vi "Test VI 1.vi"() -> ()   [LabVIEW 2022 SP3]
doc: "Block Diagram 1\n\nLorem ipsum dolor sit amet, consectetur adipiscing elit. Pellentesque gravida dolor et ex feugiat finibus."
panel:
  out "VI Description":string
  # "Front Panel 1\n\nLorem ipsum dolor sit amet, consectetur adipiscing elit. Pellentesque gravida dolor et ex feugiat finibus."
  # "Front Panel 4\n\nLorem ipsum dolor sit amet, consectetur adipiscing elit. Fusce sed augue venenatis lacus tempor malesuada. Ut eget leo sed enim aliquam porta vel at lectus. Vestibulum pretium lacinia finibus. Ut rutrum tincidunt justo, quis accumsan mauris consectetur blandit. Pellentesque sodales urna ac elit pharetra imperdiet. Phasellus felis mi, mollis non elementum et, auctor sit amet ligula. Vivamus vel dictum mi.\n\nDonec tempus orci vitae quam venenatis gravida. Nunc consequat ligula placerat ante molestie iaculis. Integer condimentum eget sapien vel vulputate. Morbi placerat, nibh iaculis gravida luctus, neque magna sodales arcu, non pellentesque mauris dolor at neque. Quisque ut erat tellus. Pellentesque nec gravida diam. Aliquam in ligula augue. Cras in tortor a erat vehicula ullamcorper ut in nisl. Nam nunc turpis, finibus id gravida vitae, interdum in dolor. Vestibulum et libero mi. Nam rhoncus lorem vulputate sodales accumsan.\n\nPhasellus in porttitor urna. Donec sodales imperdiet tellus, at interdum dolor auctor vehicula. Nullam risus sem, tincidunt ullamcorper purus nec, sagittis pharetra sem. Suspendisse blandit mattis quam et tristique. Aenean interdum quam non ligula faucibus pretium in nec ante. Curabitur euismod enim ac faucibus facilisis. Sed sed nisl finibus eros venenatis ornare sit amet quis eros. Integer pellentesque non ligula eget gravida. Aenean fringilla tempus rutrum. Nulla ullamcorper vel lacus quis sodales. Curabitur vel porttitor arcu.\n\nNam in mi sagittis, pretium eros nec, hendrerit neque. Mauris volutpat sem ut eros ornare mattis. Pellentesque at feugiat turpis. Morbi ut diam eget eros fermentum pharetra. Phasellus dictum aliquet est, vel auctor nisi. Duis eget dolor lacus. Phasellus non aliquam risus. Quisque iaculis nibh eget feugiat volutpat. Cras id augue sit amet ipsum cursus dictum a in urna.\n\nOrci varius natoque penatibus et magnis dis parturient montes, nascetur ridiculus mus. Donec id urna rhoncus, finibus orci vel, lacinia neque. Curabitur vitae semper erat. In a urna ac nisi ornare blandit non ut dolor. Nunc eu dignissim quam. Donec eros quam, vulputate vel fermentum sit amet, blandit eget nibh. Donec ut dictum sem. Nullam sed tortor eget nibh maximus dapibus. Aliquam erat volutpat. Nam a nisi sit amet diam ornare volutpat non eu ligula. Praesent ipsum enim, ullamcorper quis ullamcorper ut, euismod eu lorem. Orci varius natoque penatibus et magnis dis parturient montes, nascetur ridiculus mus. Integer condimentum id risus vitae aliquam. Nunc congue tempor ante, sit amet malesuada urna laoreet vel. Morbi dapibus tortor sapien, vel aliquet ligula egestas in.\n\nSuspendisse risus felis, tristique eu luctus in, pharetra id nunc. Aenean fringilla tellus in nisi condimentum, a faucibus odio consectetur. Fusce consectetur malesuada viverra. Nulla ante ante, facilisis et consequat vitae, eleifend sit amet lorem. Etiam hendrerit, quam in pulvinar condimentum, nibh dui dignissim est, ac viverra ipsum lorem sit amet urna. Etiam in malesuada risus. Morbi elementum interdum eleifend. Morbi sit amet est augue. Nam lobortis, orci a hendrerit scelerisque, diam odio consectetur diam, id lobortis tortor ex eget risus. Morbi enim ipsum, imperdiet quis aliquam a, molestie a ex. Sed metus eros, auctor tincidunt rutrum nec, suscipit non nunc. Aliquam vitae fermentum libero. \n\n(6 paragraphs, 500 words, 3328 bytes)"
  # "Front Panel 5\n\nLorem ipsum dolor sit amet, consectetur adipiscing elit. Sed lobortis magna ac porttitor varius. Quisque a mattis est. Suspendisse posuere tortor ut justo congue mollis. Donec odio enim, bibendum ac elit a, dictum congue neque. Maecenas in finibus ligula. Pellentesque nibh odio, fringilla placerat auctor id, tincidunt sed enim. Ut viverra metus eget vestibulum sagittis. Ut vestibulum quam at porta tincidunt. Suspendisse nisl neque, iaculis non egestas maximus, laoreet eu metus. Aenean vitae fringilla tellus, quis rutrum nisi.\n\nCurabitur eget nunc at orci aliquam dapibus quis lobortis elit. Nam sagittis velit euismod ipsum feugiat, vitae dignissim mi finibus. Pellentesque vehicula felis ante, in pellentesque odio auctor et. Aenean ultricies mollis risus, vehicula dictum eros laoreet a. Suspendisse potenti. Quisque pretium tortor eu massa ultricies iaculis. Nulla auctor tincidunt tortor a egestas. Vivamus et mauris id enim auctor semper. Ut viverra turpis id urna commodo, blandit volutpat neque consequat. Sed pharetra ex sed imperdiet pharetra. Pellentesque pharetra dui in purus pellentesque posuere. Nullam nec laoreet erat.\n\nProin non nunc rutrum, eleifend lectus non, laoreet augue. Sed commodo neque et ultrices venenatis. Aenean placerat euismod viverra. Nullam nec interdum nulla, non tristique nibh. Sed sit amet pellentesque diam. Donec porta metus sit amet leo tincidunt, et laoreet arcu suscipit. In sodales risus quis ligula consectetur, at pellentesque erat interdum. Etiam ac ipsum augue.\n\nNam aliquet et risus quis laoreet. Sed malesuada libero congue est eleifend tempus. Nullam neque justo, lobortis eget elit vitae, bibendum commodo neque. Etiam eget faucibus mi. Nunc non est urna. Proin varius ornare neque vitae pulvinar. Nulla facilisi. Aliquam diam magna, efficitur quis nibh quis, rhoncus semper libero. Sed placerat nulla urna, vel posuere ipsum eleifend vitae. Vestibulum convallis neque eu ligula mollis posuere.\n\nSed dapibus fermentum metus. Aenean vitae mollis ligula. Vestibulum sed velit massa. Sed eget tempor ex, vitae rutrum velit. Nam at dignissim libero, a blandit turpis. Nam varius accumsan tellus, non dictum lacus molestie nec. Nunc euismod ultricies cursus. Vestibulum laoreet mi vitae venenatis commodo. Vestibulum congue erat vitae sem malesuada pretium. Nam fermentum lorem at tellus varius porttitor.\n\nVestibulum viverra ex sit amet sem posuere, nec feugiat sem aliquam. Praesent dolor augue, rutrum vel quam ac, pretium mattis odio. Praesent urna risus, semper at eros non, interdum sagittis nunc. Maecenas eu diam a magna tincidunt interdum ac a tortor. Maecenas porta lacus a nisl pharetra, ut vulputate dui pretium. Nullam odio neque, aliquam ut consectetur non, ullamcorper non dolor. Duis tincidunt risus nec ipsum rutrum, viverra euismod lacus tincidunt. Suspendisse pulvinar orci vel neque facilisis tempus. Donec malesuada aliquet mattis.\n\nSed vestibulum laoreet maximus. Proin tortor nibh, sodales eu feugiat eu, commodo laoreet orci. Proin venenatis ante ipsum, nec pharetra lacus ultrices eget. Aliquam quis augue ligula. Cras non purus vitae nisl elementum eleifend id a augue. Phasellus sed justo non neque commodo varius. Duis at egestas ex. Fusce at rutrum risus. Morbi ac turpis pharetra, commodo diam nec, egestas ex. Pellentesque ipsum enim, dictum eget nunc eget, sodales sollicitudin purus. Nam bibendum auctor ante sit amet luctus. Nulla feugiat pretium tellus, interdum vulputate sem rhoncus ac. Sed tincidunt, eros vel sollicitudin vestibulum, ante felis interdum nunc, ac gravida turpis odio eget neque. Quisque consequat nibh leo. Praesent quis magna consequat, ultrices nulla id, dignissim purus. Ut suscipit, leo id malesuada tincidunt, diam velit sollicitudin ipsum, eu vehicula ipsum ipsum quis urna.\n\nSuspendisse in fermentum ante, eget eleifend odio. Sed suscipit sollicitudin nunc, at iaculis est molestie sit amet. Nulla vel tempus ligula. Morbi at nunc sed magna vehicula aliquet. Donec vitae tincidunt leo. Curabitur maximus mauris in dignissim posuere. Nunc faucibus id erat non tincidunt. Integer pellentesque nulla ut sapien fermentum sagittis.\n\nFusce mollis sodales mattis. Nunc fringilla fermentum justo, eu imperdiet erat pharetra vehicula. Sed volutpat urna lacus, at volutpat nisl bibendum vel. Quisque a augue sit amet felis luctus consequat. Nunc id imperdiet risus. Integer eros libero, semper eu erat ac, dictum tincidunt ex. Proin sit amet porta velit, at tincidunt nibh. Proin condimentum auctor lorem, vel accumsan nunc commodo a.\n\nVivamus bibendum scelerisque arcu, vitae hendrerit leo iaculis nec. Suspendisse potenti. Morbi a eros laoreet, malesuada nisi suscipit, congue nunc. Fusce imperdiet risus leo. Nunc dui magna, semper placerat elit ac, maximus venenatis felis. Curabitur luctus lobortis ante vitae tempus. Vivamus porttitor sed eros at congue.\n\nUt eu eleifend dui. Maecenas nec est suscipit, ornare urna in, laoreet magna. Aenean facilisis varius lectus, sed sodales ante facilisis quis. Vestibulum condimentum dolor venenatis posuere lobortis. Praesent dictum laoreet metus id dictum. Nulla elementum ligula eget ornare pretium. Donec sodales enim nibh, sit amet mattis ex condimentum a. Curabitur in placerat lectus. Proin viverra nec tortor id feugiat.\n\nProin eu eleifend mauris, ut fringilla tortor. Cras dapibus dolor sit amet purus iaculis porta. Vestibulum vitae ante libero. Proin tempus convallis erat, eu condimentum dui volutpat sed. Vivamus convallis pellentesque lorem ut posuere. Etiam porttitor ultricies justo nec dignissim. Phasellus leo ex, porta et vehicula et, fermentum eu neque. Pellentesque elit lorem, semper at tellus in, interdum dictum elit. Cras bibendum suscipit velit, vel rhoncus mi venenatis vel. Aenean placerat a risus eget porta. Nullam ornare odio vel interdum rhoncus. Nulla non viverra odio. \n\n(12 paragraphs, 862 words, 5830 bytes)"
  # "Front Panel 6"
  # "7"
  # "Front Panel 2\n\nLorem ipsum dolor sit amet, consectetur adipiscing elit. Pellentesque gravida dolor et ex feugiat finibus. Nullam quam nibh, venenatis ut tortor ut, blandit interdum erat. Pellentesque elementum tristique risus, et consequat sapien rutrum a. Mauris sollicitudin efficitur eros, sit amet imperdiet lectus tincidunt eget. Donec fringilla dui pharetra nulla posuere, quis semper felis venenatis. Etiam eros diam, laoreet vel rhoncus vel, lobortis ut nibh. Duis pretium pulvinar efficitur. Vivamus maximus orci sed rhoncus ornare. Nullam scelerisque mi nunc, et interdum erat dictum at. Ut a nibh in diam ornare vestibulum. Vestibulum et diam non metus pulvinar consectetur. Morbi eleifend semper velit, ac porta ex dapibus at. In sed enim nec ex aliquam fringilla non non ex. Donec faucibus sodales velit, vel gravida enim scelerisque non."
  # "Front Panel 3\n\nLorem ipsum dolor sit amet, consectetur adipiscing elit. Pellentesque gravida dolor et ex feugiat finibus. Nullam quam nibh, venenatis ut tortor ut, blandit interdum erat. Pellentesque elementum tristique risus, et consequat sapien rutrum a. Mauris sollicitudin efficitur eros, sit amet imperdiet lectus tincidunt eget. Donec fringilla dui pharetra nulla posuere, quis semper felis venenatis. Etiam eros diam, laoreet vel rhoncus vel, lobortis ut nibh. Duis pretium pulvinar efficitur. Vivamus maximus orci sed rhoncus ornare. Nullam scelerisque mi nunc, et interdum erat dictum at. Ut a nibh in diam ornare vestibulum. Vestibulum et diam non metus pulvinar consectetur. Morbi eleifend semper velit, ac porta ex dapibus at. In sed enim nec ex aliquam fringilla non non ex. Donec faucibus sodales velit, vel gravida enim scelerisque non.\n\nVivamus sagittis dignissim diam, sed rutrum purus interdum eu. Quisque posuere porttitor risus vel pellentesque. Sed quis quam pretium velit cursus convallis. Phasellus eget tellus at lorem maximus pretium. Sed fringilla sapien vel dui ornare tristique. Quisque bibendum tempus arcu a pharetra. Donec eu posuere purus. Vivamus nec pulvinar metus, vehicula mattis nulla. Mauris suscipit nulla non congue pulvinar. Donec varius magna ac euismod scelerisque. Maecenas tempus scelerisque ligula, in rutrum mi sollicitudin nec. Mauris tristique ante metus, ut lacinia est tempor sit amet. Etiam tempor pretium elit, at aliquet nisi gravida nec. Vestibulum imperdiet, ex eget ullamcorper lacinia, augue libero malesuada augue, eget porta lacus lacus vitae dolor.\n\nNunc gravida lacus nec mattis malesuada. In sem metus, eleifend eget erat quis, ornare ornare urna. Aenean varius ligula euismod semper porttitor. Donec quis justo at odio rhoncus sagittis id a nisl. Donec mollis arcu ut neque aliquam, nec pulvinar ipsum malesuada. Class aptent taciti sociosqu ad litora torquent per conubia nostra, per inceptos himenaeos. Nunc sit amet lorem quis odio laoreet rhoncus."
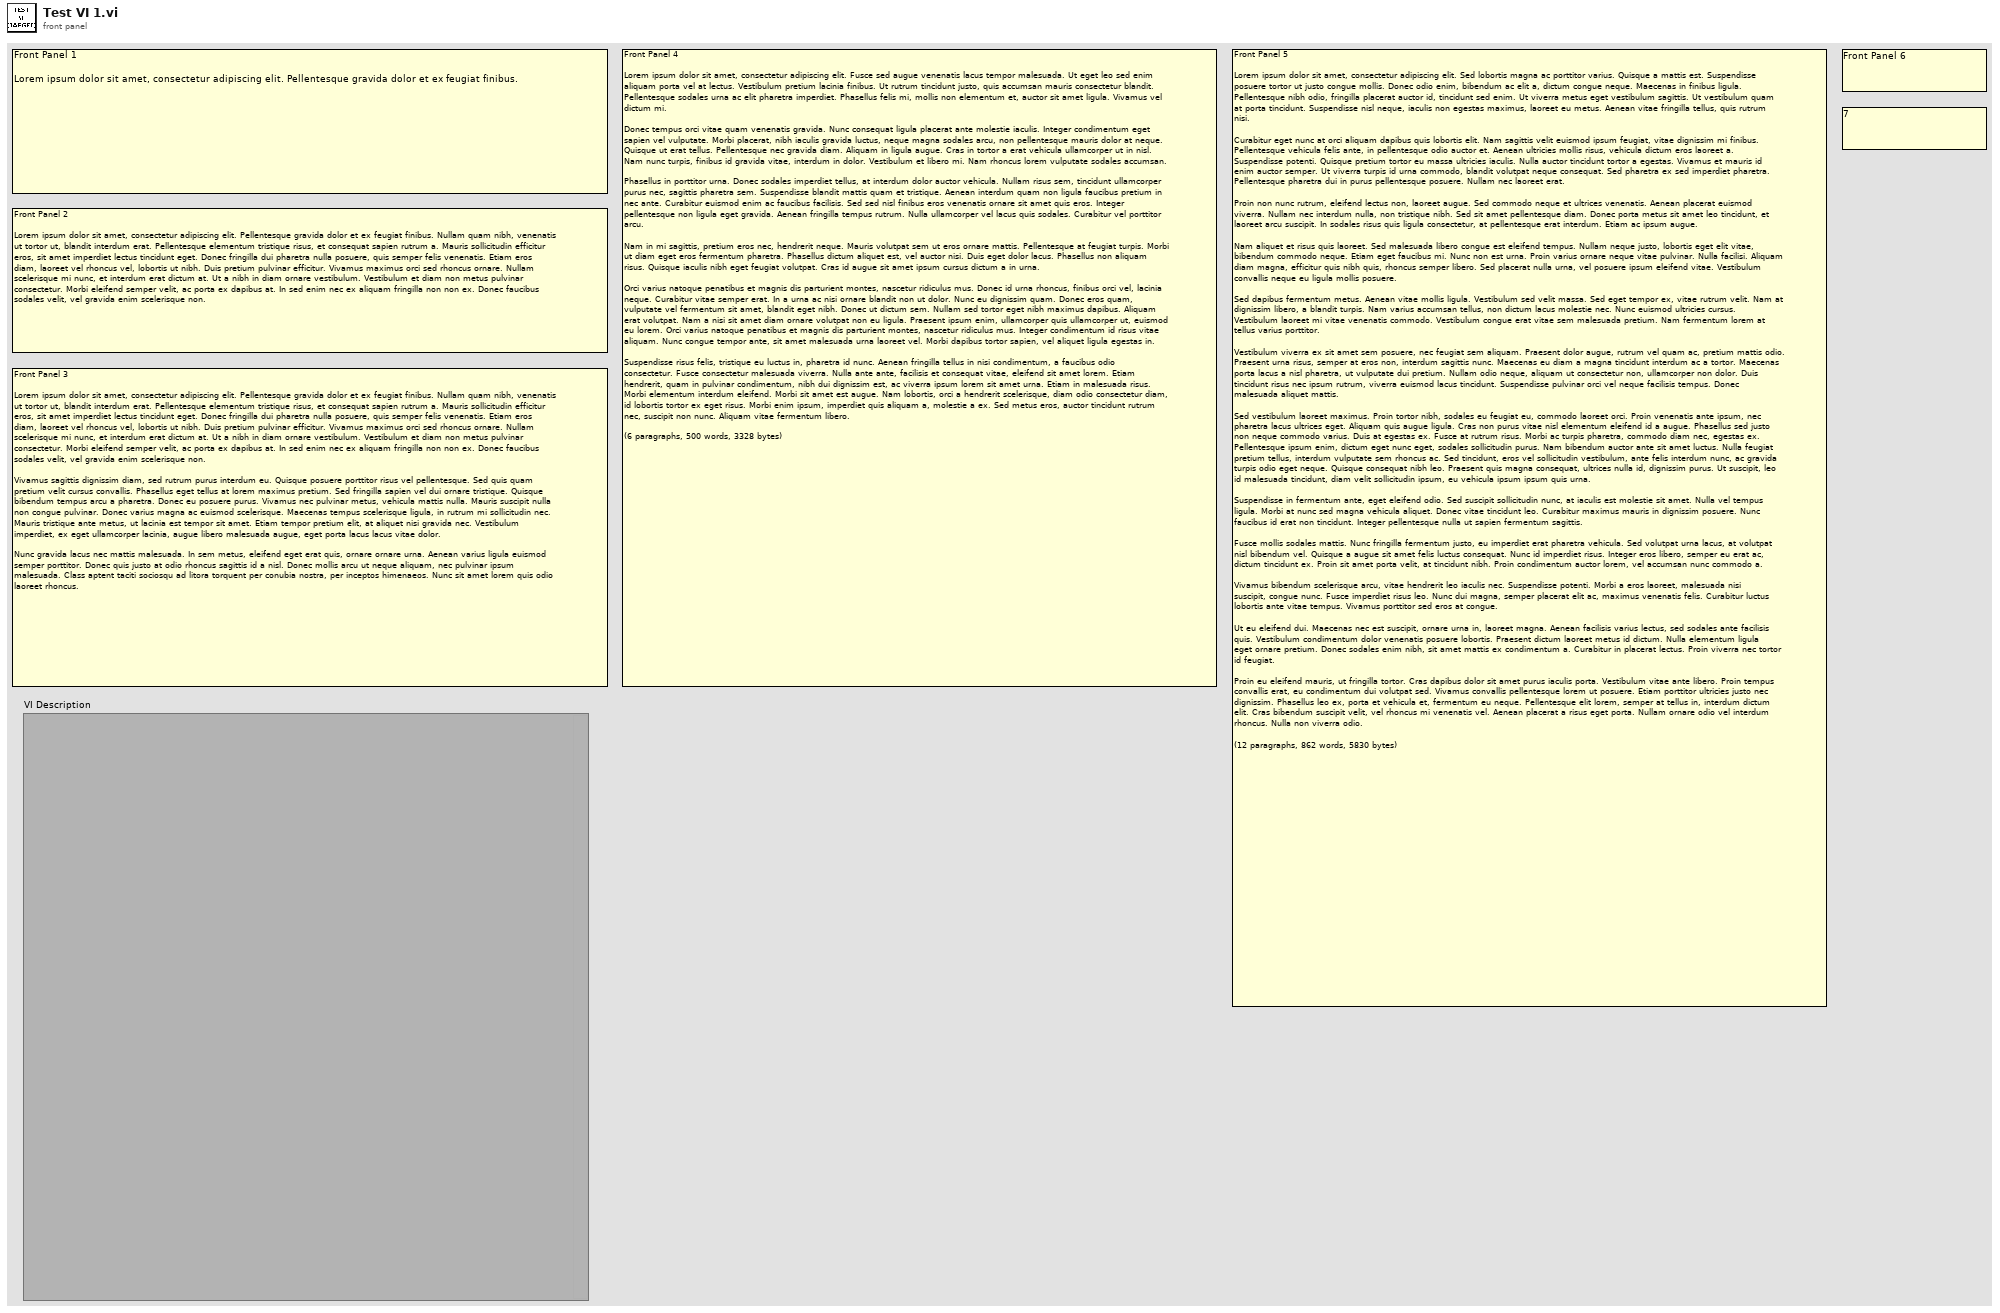
[diagram p1: front panel]
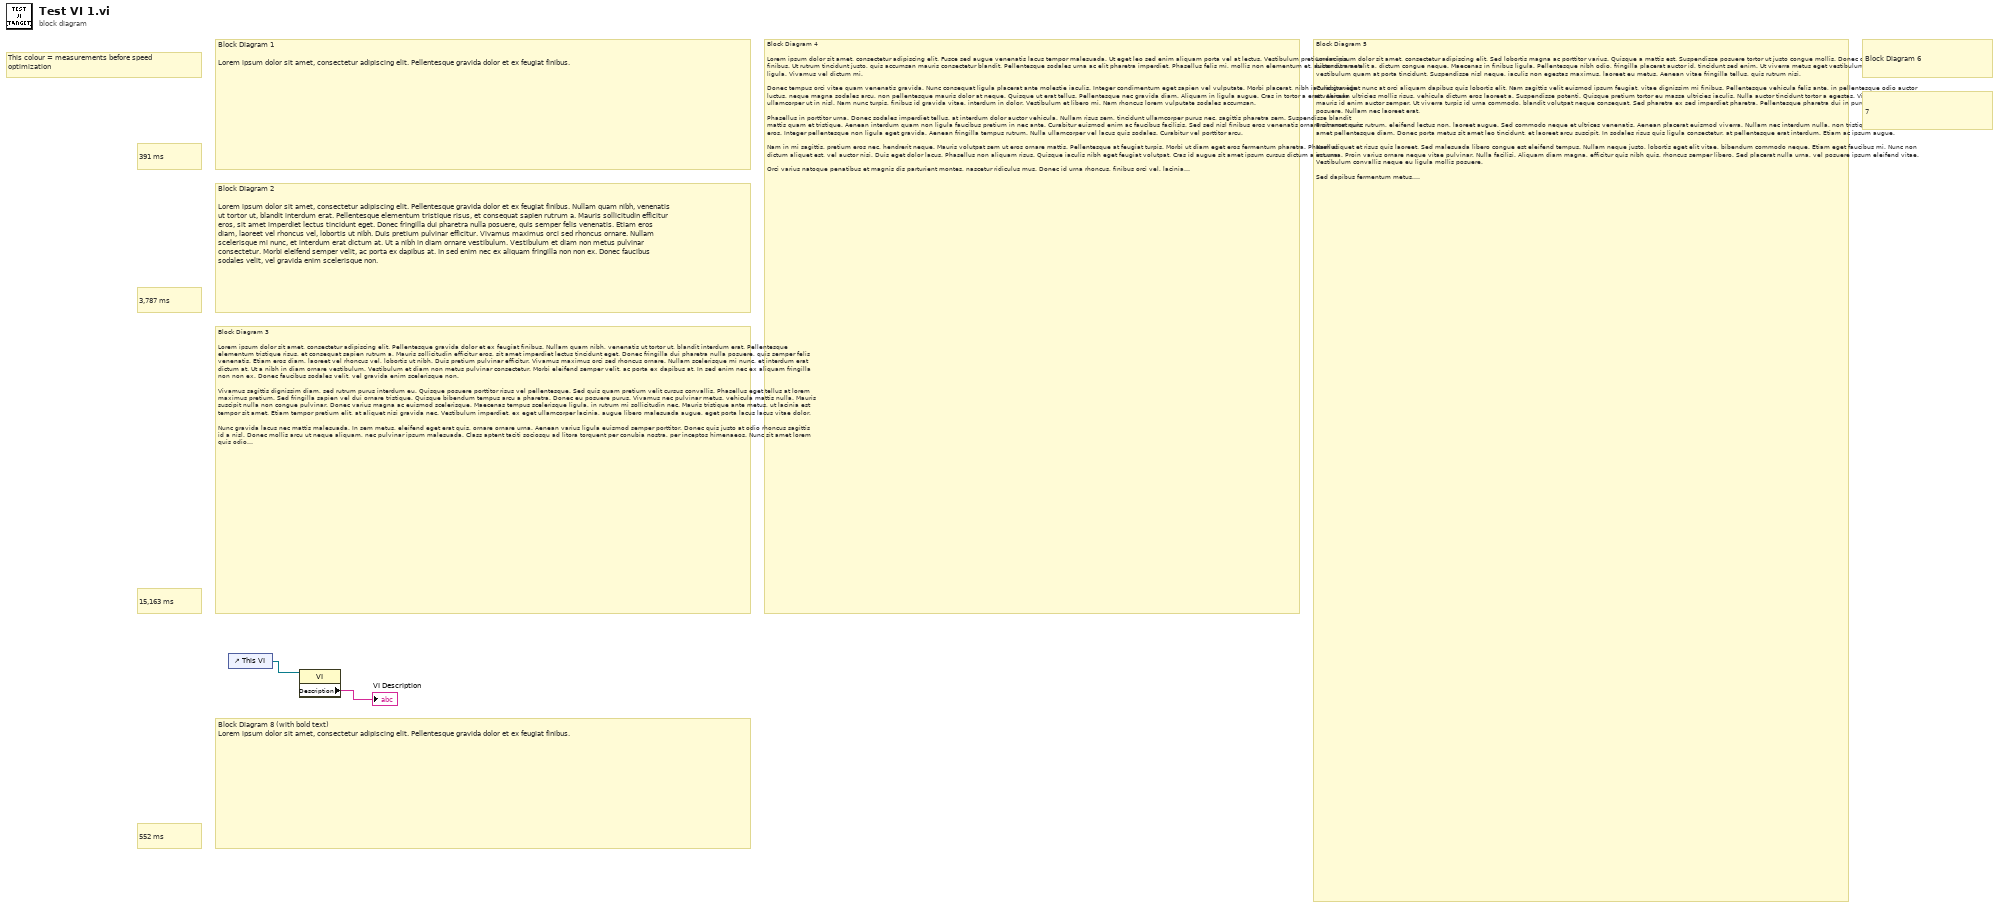
[diagram p0: block diagram]
diagram:
  # "552 ms"
  # "15,163 ms"
  # "3,787 ms"
  # "This colour = measurements before speed optimization"
  # "391 ms"
  # "Block Diagram 8 (with bold text)\nLorem ipsum dolor sit amet, consectetur adipiscing elit. Pellentesque gravida dolor et ex feugiat finibus."
  # "7"
  # "Block Diagram 6"
  # "Block Diagram 5\n\nLorem ipsum dolor sit amet, consectetur adipiscing elit. Sed lobortis magna ac porttitor varius. Quisque a mattis est. Suspendisse posuere tortor ut justo congue mollis. Donec odio enim, bibendum ac elit a, dictum congue neque. Maecenas in finibus ligula. Pellentesque nibh odio, fringilla placerat auctor id, tincidunt sed enim. Ut viverra metus eget vestibulum sagittis. Ut vestibulum quam at porta tincidunt. Suspendisse nisl neque, iaculis non egestas maximus, laoreet eu metus. Aenean vitae fringilla tellus, quis rutrum nisi.\n\nCurabitur eget nunc at orci aliquam dapibus quis lobortis elit. Nam sagittis velit euismod ipsum feugiat, vitae dignissim mi finibus. Pellentesque vehicula felis ante, in pellentesque odio auctor et. Aenean ultricies mollis risus, vehicula dictum eros laoreet a. Suspendisse potenti. Quisque pretium tortor eu massa ultricies iaculis. Nulla auctor tincidunt tortor a egestas. Vivamus et mauris id enim auctor semper. Ut viverra turpis id urna commodo, blandit volutpat neque consequat. Sed pharetra ex sed imperdiet pharetra. Pellentesque pharetra dui in purus pellentesque posuere. Nullam nec laoreet erat.\n\nProin non nunc rutrum, eleifend lectus non, laoreet augue. Sed commodo neque et ultrices venenatis. Aenean placerat euismod viverra. Nullam nec interdum nulla, non tristique nibh. Sed sit amet pellentesque diam. Donec porta metus sit amet leo tincidunt, et laoreet arcu suscipit. In sodales risus quis ligula consectetur, at pellentesque erat interdum. Etiam ac ipsum augue.\n\nNam aliquet et risus quis laoreet. Sed malesuada libero congue est eleifend tempus. Nullam neque justo, lobortis eget elit vitae, bibendum commodo neque. Etiam eget faucibus mi. Nunc non est urna. Proin varius ornare neque vitae pulvinar. Nulla facilisi. Aliquam diam magna, efficitur quis nibh quis, rhoncus semper libero. Sed placerat nulla urna, vel posuere ipsum eleifend vitae. Vestibulum convallis neque eu ligula mollis posuere.\n\nSed dapibus fermentum metus. Aenean vitae mollis ligula. Vestibulum sed velit massa. Sed eget tempor ex, vitae rutrum velit. Nam at dignissim libero, a blandit turpis. Nam varius accumsan tellus, non dictum lacus molestie nec. Nunc euismod ultricies cursus. Vestibulum laoreet mi vitae venenatis commodo. Vestibulum congue erat vitae sem malesuada pretium. Nam fermentum lorem at tellus varius porttitor.\n\nVestibulum viverra ex sit amet sem posuere, nec feugiat sem aliquam. Praesent dolor augue, rutrum vel quam ac, pretium mattis odio. Praesent urna risus, semper at eros non, interdum sagittis nunc. Maecenas eu diam a magna tincidunt interdum ac a tortor. Maecenas porta lacus a nisl pharetra, ut vulputate dui pretium. Nullam odio neque, aliquam ut consectetur non, ullamcorper non dolor. Duis tincidunt risus nec ipsum rutrum, viverra euismod lacus tincidunt. Suspendisse pulvinar orci vel neque facilisis tempus. Donec malesuada aliquet mattis.\n\nSed vestibulum laoreet maximus. Proin tortor nibh, sodales eu feugiat eu, commodo laoreet orci. Proin venenatis ante ipsum, nec pharetra lacus ultrices eget. Aliquam quis augue ligula. Cras non purus vitae nisl elementum eleifend id a augue. Phasellus sed justo non neque commodo varius. Duis at egestas ex. Fusce at rutrum risus. Morbi ac turpis pharetra, commodo diam nec, egestas ex. Pellentesque ipsum enim, dictum eget nunc eget, sodales sollicitudin purus. Nam bibendum auctor ante sit amet luctus. Nulla feugiat pretium tellus, interdum vulputate sem rhoncus ac. Sed tincidunt, eros vel sollicitudin vestibulum, ante felis interdum nunc, ac gravida turpis odio eget neque. Quisque consequat nibh leo. Praesent quis magna consequat, ultrices nulla id, dignissim purus. Ut suscipit, leo id malesuada tincidunt, diam velit sollicitudin ipsum, eu vehicula ipsum ipsum quis urna.\n\nSuspendisse in fermentum ante, eget eleifend odio. Sed suscipit sollicitudin nunc, at iaculis est molestie sit amet. Nulla vel tempus ligula. Morbi at nunc sed magna vehicula aliquet. Donec vitae tincidunt leo. Curabitur maximus mauris in dignissim posuere. Nunc faucibus id erat non tincidunt. Integer pellentesque nulla ut sapien fermentum sagittis.\n\nFusce mollis sodales mattis. Nunc fringilla fermentum justo, eu imperdiet erat pharetra vehicula. Sed volutpat urna lacus, at volutpat nisl bibendum vel. Quisque a augue sit amet felis luctus consequat. Nunc id imperdiet risus. Integer eros libero, semper eu erat ac, dictum tincidunt ex. Proin sit amet porta velit, at tincidunt nibh. Proin condimentum auctor lorem, vel accumsan nunc commodo a.\n\nVivamus bibendum scelerisque arcu, vitae hendrerit leo iaculis nec. Suspendisse potenti. Morbi a eros laoreet, malesuada nisi suscipit, congue nunc. Fusce imperdiet risus leo. Nunc dui magna, semper placerat elit ac, maximus venenatis felis. Curabitur luctus lobortis ante vitae tempus. Vivamus porttitor sed eros at congue.\n\nUt eu eleifend dui. Maecenas nec est suscipit, ornare urna in, laoreet magna. Aenean facilisis varius lectus, sed sodales ante facilisis quis. Vestibulum condimentum dolor venenatis posuere lobortis. Praesent dictum laoreet metus id dictum. Nulla elementum ligula eget ornare pretium. Donec sodales enim nibh, sit amet mattis ex condimentum a. Curabitur in placerat lectus. Proin viverra nec tortor id feugiat.\n\nProin eu eleifend mauris, ut fringilla tortor. Cras dapibus dolor sit amet purus iaculis porta. Vestibulum vitae ante libero. Proin tempus convallis erat, eu condimentum dui volutpat sed. Vivamus convallis pellentesque lorem ut posuere. Etiam porttitor ultricies justo nec dignissim. Phasellus leo ex, porta et vehicula et, fermentum eu neque. Pellentesque elit lorem, semper at tellus in, interdum dictum elit. Cras bibendum suscipit velit, vel rhoncus mi venenatis vel. Aenean placerat a risus eget porta. Nullam ornare odio vel interdum rhoncus. Nulla non viverra odio. \n\n(12 paragraphs, 862 words, 5830 bytes)"
  # "Block Diagram 4\n\nLorem ipsum dolor sit amet, consectetur adipiscing elit. Fusce sed augue venenatis lacus tempor malesuada. Ut eget leo sed enim aliquam porta vel at lectus. Vestibulum pretium lacinia finibus. Ut rutrum tincidunt justo, quis accumsan mauris consectetur blandit. Pellentesque sodales urna ac elit pharetra imperdiet. Phasellus felis mi, mollis non elementum et, auctor sit amet ligula. Vivamus vel dictum mi.\n\nDonec tempus orci vitae quam venenatis gravida. Nunc consequat ligula placerat ante molestie iaculis. Integer condimentum eget sapien vel vulputate. Morbi placerat, nibh iaculis gravida luctus, neque magna sodales arcu, non pellentesque mauris dolor at neque. Quisque ut erat tellus. Pellentesque nec gravida diam. Aliquam in ligula augue. Cras in tortor a erat vehicula ullamcorper ut in nisl. Nam nunc turpis, finibus id gravida vitae, interdum in dolor. Vestibulum et libero mi. Nam rhoncus lorem vulputate sodales accumsan.\n\nPhasellus in porttitor urna. Donec sodales imperdiet tellus, at interdum dolor auctor vehicula. Nullam risus sem, tincidunt ullamcorper purus nec, sagittis pharetra sem. Suspendisse blandit mattis quam et tristique. Aenean interdum quam non ligula faucibus pretium in nec ante. Curabitur euismod enim ac faucibus facilisis. Sed sed nisl finibus eros venenatis ornare sit amet quis eros. Integer pellentesque non ligula eget gravida. Aenean fringilla tempus rutrum. Nulla ullamcorper vel lacus quis sodales. Curabitur vel porttitor arcu.\n\nNam in mi sagittis, pretium eros nec, hendrerit neque. Mauris volutpat sem ut eros ornare mattis. Pellentesque at feugiat turpis. Morbi ut diam eget eros fermentum pharetra. Phasellus dictum aliquet est, vel auctor nisi. Duis eget dolor lacus. Phasellus non aliquam risus. Quisque iaculis nibh eget feugiat volutpat. Cras id augue sit amet ipsum cursus dictum a in urna.\n\nOrci varius natoque penatibus et magnis dis parturient montes, nascetur ridiculus mus. Donec id urna rhoncus, finibus orci vel, lacinia neque. Curabitur vitae semper erat. In a urna ac nisi ornare blandit non ut dolor. Nunc eu dignissim quam. Donec eros quam, vulputate vel fermentum sit amet, blandit eget nibh. Donec ut dictum sem. Nullam sed tortor eget nibh maximus dapibus. Aliquam erat volutpat. Nam a nisi sit amet diam ornare volutpat non eu ligula. Praesent ipsum enim, ullamcorper quis ullamcorper ut, euismod eu lorem. Orci varius natoque penatibus et magnis dis parturient montes, nascetur ridiculus mus. Integer condimentum id risus vitae aliquam. Nunc congue tempor ante, sit amet malesuada urna laoreet vel. Morbi dapibus tortor sapien, vel aliquet ligula egestas in.\n\nSuspendisse risus felis, tristique eu luctus in, pharetra id nunc. Aenean fringilla tellus in nisi condimentum, a faucibus odio consectetur. Fusce consectetur malesuada viverra. Nulla ante ante, facilisis et consequat vitae, eleifend sit amet lorem. Etiam hendrerit, quam in pulvinar condimentum, nibh dui dignissim est, ac viverra ipsum lorem sit amet urna. Etiam in malesuada risus. Morbi elementum interdum eleifend. Morbi sit amet est augue. Nam lobortis, orci a hendrerit scelerisque, diam odio consectetur diam, id lobortis tortor ex eget risus. Morbi enim ipsum, imperdiet quis aliquam a, molestie a ex. Sed metus eros, auctor tincidunt rutrum nec, suscipit non nunc. Aliquam vitae fermentum libero. \n\n(6 paragraphs, 500 words, 3328 bytes)"
  # "Block Diagram 3\n\nLorem ipsum dolor sit amet, consectetur adipiscing elit. Pellentesque gravida dolor et ex feugiat finibus. Nullam quam nibh, venenatis ut tortor ut, blandit interdum erat. Pellentesque elementum tristique risus, et consequat sapien rutrum a. Mauris sollicitudin efficitur eros, sit amet imperdiet lectus tincidunt eget. Donec fringilla dui pharetra nulla posuere, quis semper felis venenatis. Etiam eros diam, laoreet vel rhoncus vel, lobortis ut nibh. Duis pretium pulvinar efficitur. Vivamus maximus orci sed rhoncus ornare. Nullam scelerisque mi nunc, et interdum erat dictum at. Ut a nibh in diam ornare vestibulum. Vestibulum et diam non metus pulvinar consectetur. Morbi eleifend semper velit, ac porta ex dapibus at. In sed enim nec ex aliquam fringilla non non ex. Donec faucibus sodales velit, vel gravida enim scelerisque non.\n\nVivamus sagittis dignissim diam, sed rutrum purus interdum eu. Quisque posuere porttitor risus vel pellentesque. Sed quis quam pretium velit cursus convallis. Phasellus eget tellus at lorem maximus pretium. Sed fringilla sapien vel dui ornare tristique. Quisque bibendum tempus arcu a pharetra. Donec eu posuere purus. Vivamus nec pulvinar metus, vehicula mattis nulla. Mauris suscipit nulla non congue pulvinar. Donec varius magna ac euismod scelerisque. Maecenas tempus scelerisque ligula, in rutrum mi sollicitudin nec. Mauris tristique ante metus, ut lacinia est tempor sit amet. Etiam tempor pretium elit, at aliquet nisi gravida nec. Vestibulum imperdiet, ex eget ullamcorper lacinia, augue libero malesuada augue, eget porta lacus lacus vitae dolor.\n\nNunc gravida lacus nec mattis malesuada. In sem metus, eleifend eget erat quis, ornare ornare urna. Aenean varius ligula euismod semper porttitor. Donec quis justo at odio rhoncus sagittis id a nisl. Donec mollis arcu ut neque aliquam, nec pulvinar ipsum malesuada. Class aptent taciti sociosqu ad litora torquent per conubia nostra, per inceptos himenaeos. Nunc sit amet lorem quis odio laoreet rhoncus."
  # "Block Diagram 2\n\nLorem ipsum dolor sit amet, consectetur adipiscing elit. Pellentesque gravida dolor et ex feugiat finibus. Nullam quam nibh, venenatis ut tortor ut, blandit interdum erat. Pellentesque elementum tristique risus, et consequat sapien rutrum a. Mauris sollicitudin efficitur eros, sit amet imperdiet lectus tincidunt eget. Donec fringilla dui pharetra nulla posuere, quis semper felis venenatis. Etiam eros diam, laoreet vel rhoncus vel, lobortis ut nibh. Duis pretium pulvinar efficitur. Vivamus maximus orci sed rhoncus ornare. Nullam scelerisque mi nunc, et interdum erat dictum at. Ut a nibh in diam ornare vestibulum. Vestibulum et diam non metus pulvinar consectetur. Morbi eleifend semper velit, ac porta ex dapibus at. In sed enim nec ex aliquam fringilla non non ex. Donec faucibus sodales velit, vel gravida enim scelerisque non."
  # "Block Diagram 1\n\nLorem ipsum dolor sit amet, consectetur adipiscing elit. Pellentesque gravida dolor et ex feugiat finibus."
  n1 = control-ref of="This VI"() -> (w1:refnum<vi>)
  n2 = property class="VI"(reference=w1) -> ("Description"=→"VI Description":string)  [unwired: 1 in, 2 out]
